vi "get_ra_table.vi"(8 "error in (no error)":errorcluster, 11 "TrajectoryMH100122AODRAPS in":refnum<class "TrajectoryMH100122AODRAPS.lvclass">) -> (0 "error out":errorcluster, 2 "RAPS points":T1[](array[typedef]), 3 "TrajectoryMH100122AODRAPS out":refnum<class "TrajectoryMH100122AODRAPS.lvclass">)   [LabVIEW 2010, in "TrajectoryMH100122AODRAPS.lvclass"]
uses:
  TrajectoryMH100122AODRAPS.lvclass
  FPGAWrapper/FPGAWrapperMH120124AOD/FPGAWrapperMH120124RAPS_PXI7813R/raps_point_cluster.ctl
  TrajectoryMH100122AODRAPS.lvclass/TrajectoryMH100122AODRAPS.ctl
  FPGAWrapper/FPGAWrapperMH120124AOD/FPGAWrapperMH120124RAPS_PXI7813R/FPGAWrapperMH120124RAPS_PXI7813R.lvclass
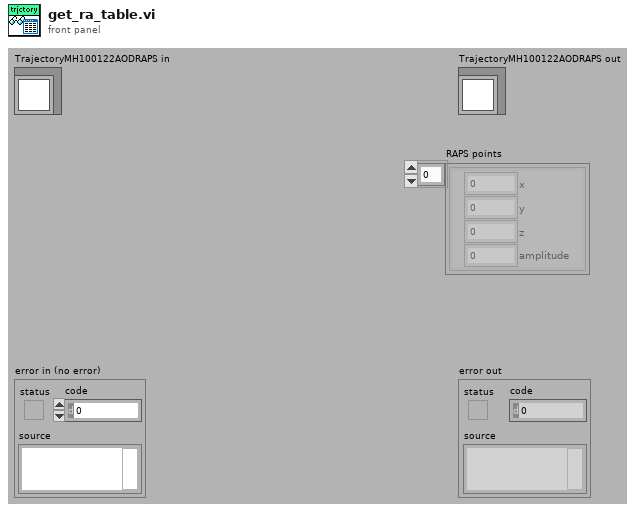
[diagram p1: front panel]
types:
  T1 = typedef "FPGAWrapperMH120124RAPS_PXI7813R.lvclass/raps_point_cluster.ctl" = cluster{"x":u16, "y":u16, "z":u16, "amplitude":u16}
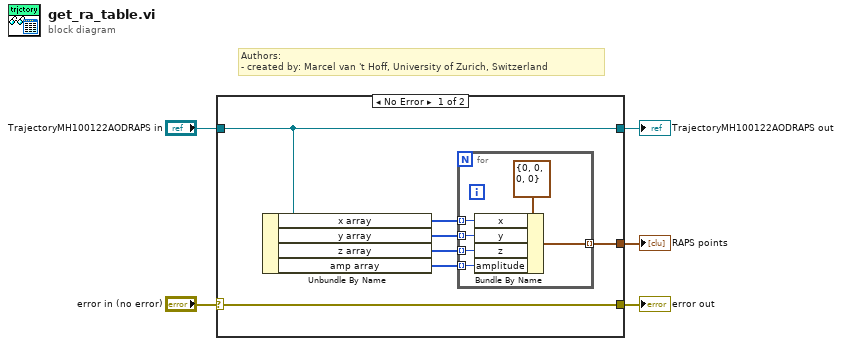
[diagram p0: block diagram]
diagram:
  # "Authors: \n- created by: Marcel van 't Hoff, University of Zurich, Switzerland"
  n1 = case shown="No Error" "error in (no error)" {
    selector: "error in (no error)" -> [w12 w20]
    tunnel: [w12 w20] -> w4
    tunnel: [w11 w19] -> w2
    tunnel: "TrajectoryMH100122AODRAPS in" -> [w11 w19]
    tunnel: [w6 _] -> w1
    frame No Error {
      n2 = Unbundle By Name(w11) -> ("x array"=w10:u16[], "y array"=w9:u16[], "z array"=w8:u16[], "amp array"=w7:u16[])
      n3 = for {
        tunnel: w10 -> [w17] mode=indexing
        tunnel: w9 -> [w16] mode=indexing
        tunnel: w8 -> [w15] mode=indexing
        tunnel: w7 -> [w14] mode=indexing
        tunnel: [w13] -> w6 mode=indexing
        n4 = Bundle By Name(cluster=T1 {"x"=0, "y"=0, "z"=0, "amplitude"=0} ("RAPS point"), "x"=w17, "y"=w16, "z"=w15, "amplitude"=w14) -> (w13:T1)
      }
    }
    frame Error {
    }
  }
  "error out" <- w4
  "TrajectoryMH100122AODRAPS out" <- w2
  "RAPS points" <- w1
